vi "Lookup Ancestor.vi"(8 "error in (no error)":errorcluster, 9 "Descendant":refnum<class "Config Element.lvclass">, 10 "Lookup":refnum<class "Config Lookup.lvclass">, 11 "Config Manager in":refnum<class "Config Manager.lvclass">) -> (0 "error out":errorcluster, 2 "Ancestor":refnum<class "Config Element.lvclass">, 3 "Config Manager out":refnum<class "Config Manager.lvclass">)   [LabVIEW 2020, in "CDM-Config.lvlib" / "Config Manager.lvclass"]
doc: "Searches towards the root of the config tree from a starting element for the first element that matches the conditions configured in <b>Lookup</b>. For more information about configuring lookups read the VI descriptions of VIs in the <b>Config Lookup</b> class."
uses:
  Config Manager.lvclass
  Config Filter/Config Lookup.lvclass
  Config Element/Config Element.lvclass
  Config Element/Config Element.lvclass/Config Element.ctl
  Config Manager.lvclass/Config Manager.ctl
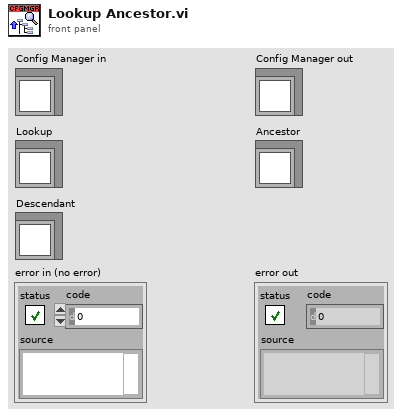
[diagram p1: front panel]
types:
  T1 = typedef "CDM-Config.lvlib/Meta Data.ctl" = cluster{"Name":string, "Value":string}
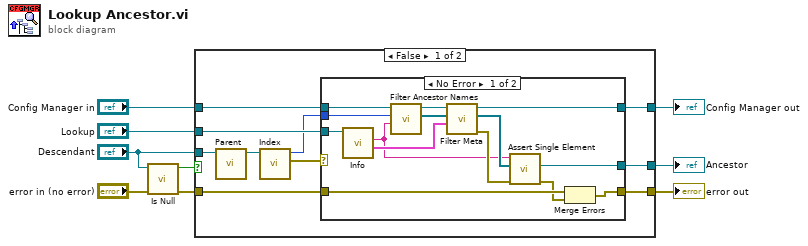
[diagram p0: block diagram]
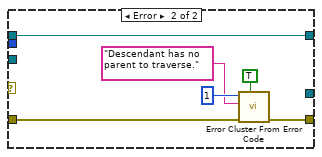
[diagram p2: hidden frame]
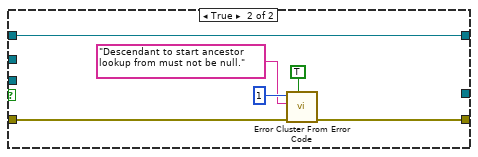
[diagram p3: hidden frame]
diagram:
  n1 = call "Is Null.vi"("Config Element in"="Descendant") -> ("Null"=w4:bool)  [unwired: 10 in]
  n2 = case shown="False" w4 {
    tunnel: "Lookup" -> [w18 _]
    tunnel: "Config Manager in" -> [w14 w40]
    tunnel: [w17 w40] -> w6
    tunnel: [w16 w43] -> w5
    tunnel: "error in (no error)" -> [w15 w44]
    tunnel: "Descendant" -> [w13 _]
    tunnel: [w9 _] -> w1
    frame False {
      n3 = call "Parent.vi"("Config Element in"=w13) -> ("Parent"=w12:refnum<class "Config Element.lvclass">)  [unwired: 9 in, 1 out]
      n4 = call "Index.vi"("Config Element in"=w12) -> ("error out"=w10:errorcluster, "Index"=w11:i32)  [unwired: 9 in]
      n5 = case shown="No Error" w10 {
        tunnel: w18 -> [w32 _]
        tunnel: [w30 w37] -> w17
        tunnel: [w29 w33] -> w16
        tunnel: w15 -> [w28 w38]
        tunnel: w14 -> [w27 w37]
        tunnel: w11 -> [w24 _]
        tunnel: [w20 _] -> w9
        frame No Error {
          n6 = call "Info.vi"("Config Lookup in"=w32) -> ("Meta"=w31:T1[], "Name"=w19:string)  [unwired: 9 in]
          n7 = call "Filter Ancestor Names.vi"("Name"=w19, "Start Index"=w24, "Config Manager in"=w27) -> ("Elements"=w25:refnum<class "Config Element.lvclass">[], "Config Manager out"=w26:refnum<class "Config Manager.lvclass">)  [unwired: 6 in, 1 out]
          n8 = call "Filter Meta.vi"("Meta"=w31, "Elements"=w25, "Config Manager in"=w26) -> ("error out"=w22:errorcluster, "Matches"=w23:refnum<class "Config Element.lvclass">[], "Config Manager out"=w30:refnum<class "Config Manager.lvclass">)  [unwired: 6 in]
          n9 = call "Assert Single Element.vi"("error in (no error)"=w22, "Elements"=w23, "Starting Name"=w19) -> ("error out"=w21:errorcluster, "Element"=w20:refnum<class "Config Element.lvclass">)  [unwired: 7 in]
          n10 = Merge Errors(w28, w21) -> (w29:errorcluster)
        }
        frame Error {
          n11 = call <vilib>:"Error Cluster From Error Code.vi"("show call chain? (False)"=TRUE, "error in (no error)"=w38, "error message (\"\")"="Descendant has no parent to traverse.", "error code (0)"=1) -> ("error out"=w33:errorcluster)  [unwired: 5 in]
        }
      }
    }
    frame True {
      n12 = call <vilib>:"Error Cluster From Error Code.vi"("show call chain? (False)"=TRUE, "error in (no error)"=w44, "error message (\"\")"="Descendant to start ancestor lookup from must not be null.", "error code (0)"=1) -> ("error out"=w43:errorcluster)  [unwired: 5 in]
    }
  }
  "error out" <- w5
  "Config Manager out" <- w6
  "Ancestor" <- w1
